vi "Calculate DNL - Code Transitions.vi"(10 "ideal code width":dbl, 11 "code transitions":dbl[](array[numeric])) -> (3 "DNL":dbl[](array[numeric]))   [LabVIEW 2021]
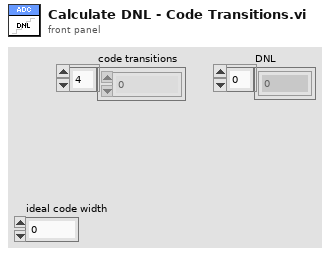
[diagram p1: front panel]
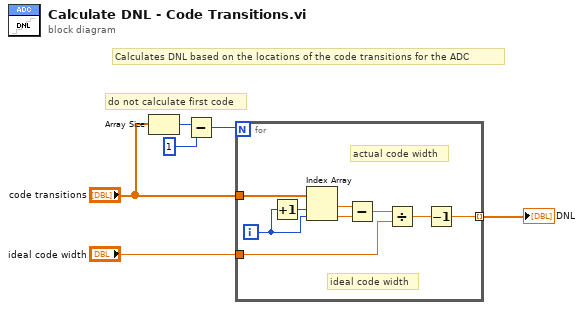
[diagram p0: block diagram]
diagram:
  # "Calculates DNL based on the locations of the code transitions for the ADC"
  # "do not calculate first code"
  n1 = Array Size(array="code transitions") -> (size(s)=w3:i32)
  n2 = Subtract(x=w3, y=1) -> (x-y=w4:i32)
  n3 = for {
    N: w4 -> [_]
    tunnel: "code transitions" -> [w15]
    tunnel: "ideal code width" -> [w9]
    tunnel: [w7] -> w6 mode=indexing
    i -> [w13]
    # "ideal code width"
    # "actual code width"
    n4 = Increment(x=w13) -> (x+1=w14:i32)
    n5 = Index Array(array=w15, index #1=w14, index #2=w13) -> (element #1=w11:dbl, element #2=w12:dbl)
    n6 = Subtract(x=w11, y=w12) -> (x-y=w10:dbl)
    n7 = Divide(x=w10, y=w9) -> (x/y=w8:dbl)
    n8 = Decrement(x=w8) -> (x-1=w7:dbl)
  }
  "DNL" <- w6
